vi "process_data.vi"(0 "Array position in":i32, 5 "Eventnum array in":i64[](array[numeric]), 7 "Polarization array in":dbl[](array[numeric]), 9 "New eventnum":i64, 11 "New polarization":dbl) -> (4 "Array position out":i32, 6 "Eventnum array out":i64[](array[numeric]), 8 "Polarization array out":dbl[](array[numeric]), 15 "Added data point":bool)   [LabVIEW 2010]
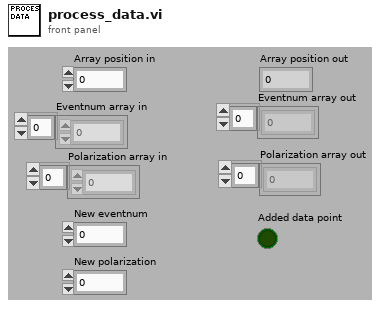
[diagram p1: front panel]
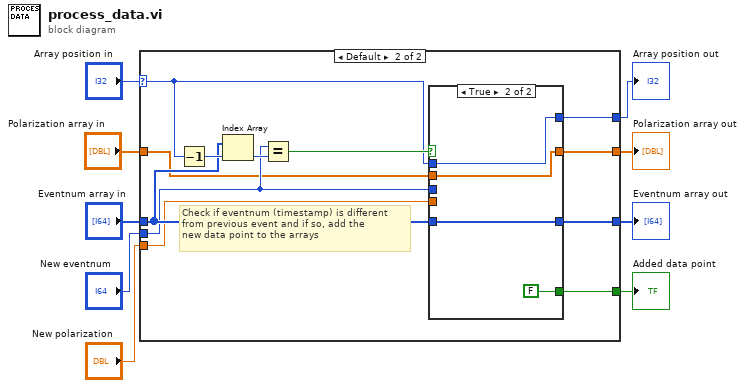
[diagram p0: block diagram]
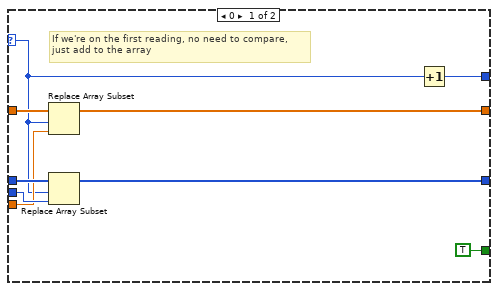
[diagram p2: hidden frame]
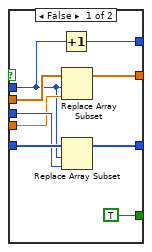
[diagram p3: hidden frame]
diagram:
  n1 = case shown="Default" "Array position in" {
    selector: "Array position in" -> [w12 w24]
    tunnel: "New eventnum" -> [w18 w25]
    tunnel: "New polarization" -> [w15 w22]
    tunnel: "Eventnum array in" -> [w17 w26]
    tunnel: "Polarization array in" -> [w14 w21]
    tunnel: [w16 w23] -> w9
    tunnel: [w13 w20] -> w8
    tunnel: [w11 w27] -> w6
    tunnel: [TRUE w19] -> w1
    frame 0 {
      # "If we're on the first reading, no need to compare,\njust add to the array"
      n2 = Replace Array Subset(array=w14, new element=w15, index=w12) -> (w13:dbl[])
      n3 = Replace Array Subset(array=w17, new element=w18, index=w12) -> (w16:i64[])
      n4 = Increment(x=w12) -> (x+1=w11:i32)
    }
    frame Default {
      # "Check if eventnum (timestamp) is different\nfrom previous event and if so, add the\nnew data point to the arrays"
      n5 = Decrement(x=w24) -> (x-1=w30:i32)
      n6 = Index Array(array=w26, index=w30) -> (element=w29:i64)
      n7 = Equal?(x=w25, y=w29) -> (x = y?=w28:bool)
      n8 = case shown="True" w28 {
        tunnel: [w32 w41] -> w27
        tunnel: w26 -> [w39 w42]
        tunnel: w25 -> [w38 _]
        tunnel: w24 -> [w33 w41]
        tunnel: [w37 w42] -> w23
        tunnel: w22 -> [w36 _]
        tunnel: w21 -> [w35 w43]
        tunnel: [w34 w43] -> w20
        tunnel: [TRUE FALSE] -> w19
        frame False {
          n9 = Increment(x=w33) -> (x+1=w32:i32)
          n10 = Replace Array Subset(array=w35, new element=w36, index=w33) -> (w34:dbl[])
          n11 = Replace Array Subset(array=w39, new element=w38, index=w33) -> (w37:i64[])
        }
        frame True {
        }
      }
    }
  }
  "Eventnum array out" <- w9
  "Polarization array out" <- w8
  "Array position out" <- w6
  "Added data point" <- w1
